vi "Kinect Extract Background 2.vi"(0 "Background Image In":T2, 1 "Depth Image In":T2, 3 "Median Filter Size":i32 min=0 max=7, 4 "Divisor":sgl=1.0 min=0 max=1 step=0.1, 5 "Distance to Camera Visible":cluster{dbl, dbl}(slide)={0.0, 32768.0} scale=-32768.0..32768.0, 6 "Post Proc Bounds":cluster{dbl, dbl}(slide)={0.0, 32768.0} scale=-3000.0..3000.0, 7 "error in":errorcluster) -> (20 "Processed Image Out":T2, 27 "error out":errorcluster)   [LabVIEW 2011]
uses:
  <vilib>/vision/Image Controls.llb/IMAQ Image.ctl
  <vilib>/vision/NI_Vision_Development_Module.lvlib
panel:
  in  "Morph Op":T1(ring)=enum."Open"
  in  "Post Proc Filter Divisor":sgl=1.0 min=0 max=1 step=0.1
  in  "Postproc Filter Size":i32 min=0 max=7
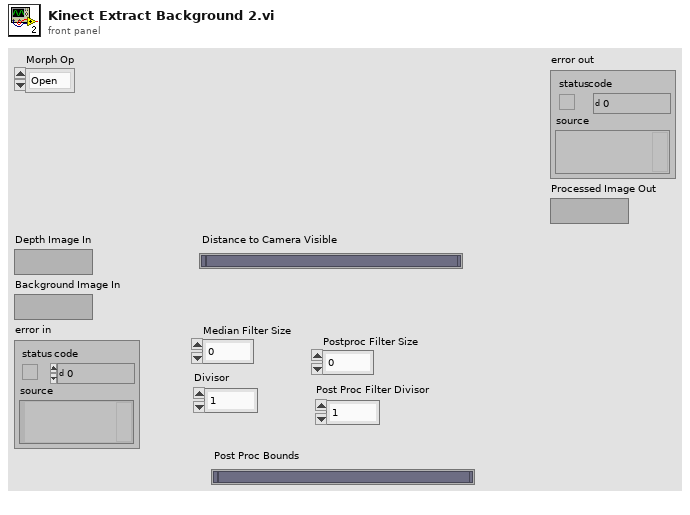
[diagram p1: front panel]
types:
  T1 = enum32{"AutoM", "Close", "Dilate", "Erode", "Gradient", "Gradient in", "Gradient out", "HitMiss", "Open", "PClose", "POpen", "Thick", "Thin"}
  T2 = typedef "IMAQ Image.ctl" = refnum<image>
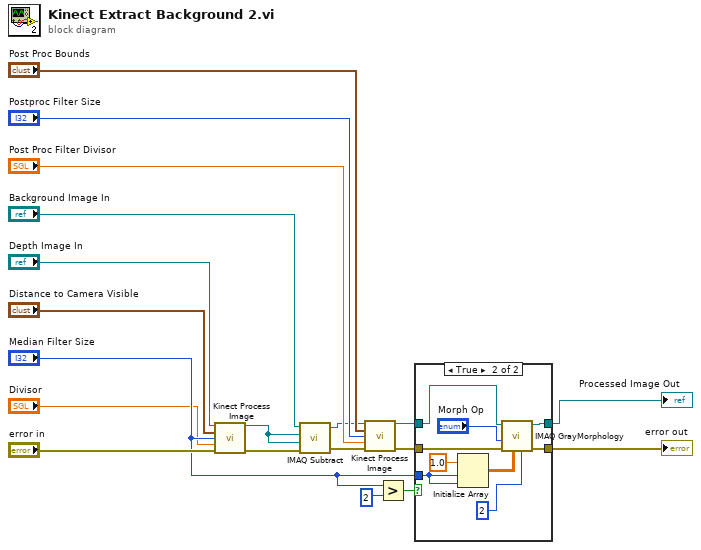
[diagram p0: block diagram]
diagram:
  n1 = call "Kinect Process Image.vi"("Depth Image In"="Depth Image In", "Distance to Camera Visible"="Distance to Camera Visible", "Median Filter Size"="Median Filter Size", "Divisor"="Divisor", "error in (no error)"="error in") -> ("Image Dst Out"=w1:T2, "error out"=w2:errorcluster)  [unwired: 9 in]
  n2 = call "IMAQ Subtract"("Image Src A"="Background Image In", "Image Dst"=w1, "Image Src B"=w1, "error in (no error)"=w2) -> ("Image Dst Out"=w3:T2, "error out"=w8:errorcluster)  [unwired: 3 in]
  n3 = call "Kinect Process Image.vi"("Depth Image In"=w3, "Distance to Camera Visible"="Post Proc Bounds", "Median Filter Size"="Postproc Filter Size", "Divisor"="Post Proc Filter Divisor", "error in (no error)"=w8) -> ("Image Dst Out"=w7:T2, "error out"=w6:errorcluster)  [unwired: 9 in]
  n4 = Greater?(x="Median Filter Size", y=2) -> (0:w4:bool)
  n5 = case shown="True" w4 {
    tunnel: w7 -> [w20 w29]
    tunnel: w6 -> [w21 w28]
    tunnel: [w21 w27] -> w13
    tunnel: [w20 w26] -> w12
    tunnel: "Median Filter Size" -> [_ w23]
    frame False {
    }
    frame True {
      n6 = Initialize Array(1.0 ("element"), w23, w23) -> (w22:dbl[][])
      n7 = call "IMAQ GrayMorphology"("Number of iterations (1)"=2, "Structuring Element"=w22, "error in (no error)"=w28, "Operation"="Morph Op", "Image Src"=w29) -> ("error out"=w27:errorcluster, "Image Dst Out"=w26:T2)  [unwired: 5 in]
    }
  }
  "error out" <- w13
  "Processed Image Out" <- w12
